vi "simpleReader.vi"() -> ()   [LabVIEW 2012]
uses:
  <userlib>/Common/Communication/ActiveMQ/ActiveMQBroker/ActiveMQBroker.lvclass
panel:
  out "messages received":string[][](table)
  in  "stopReader":bool
  in  "topic":string="testTopic"
  in  "port":string="61616"
  in  "host":string="localhost"
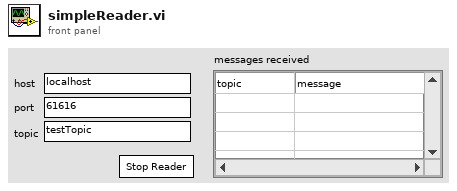
[diagram p1: front panel]
types:
  T1 = enum32{"invalid app kind", "Development System", "Run Time System", "Student Edition", "Embedded LabVIEW", "Evaluation", "Custom"}
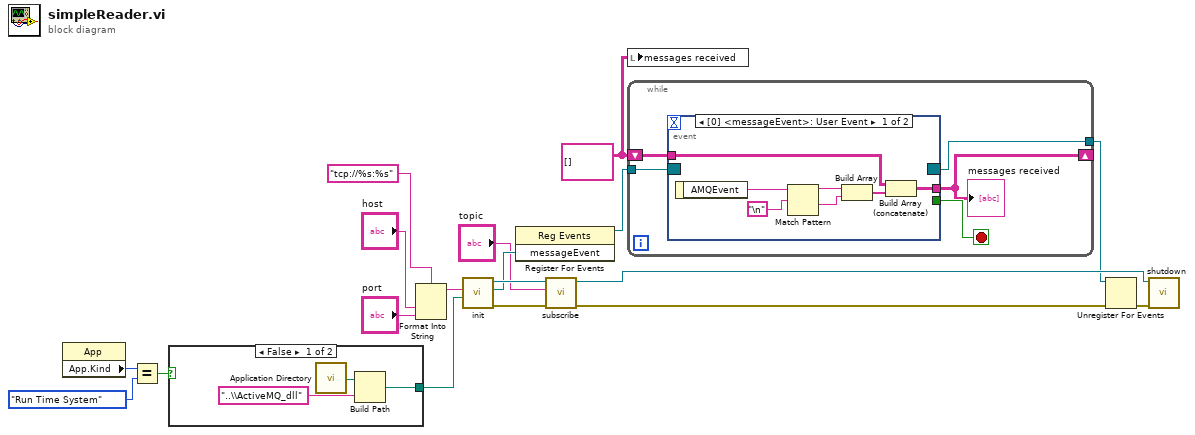
[diagram p0: block diagram]
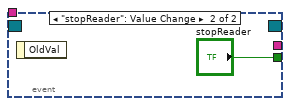
[diagram p2: hidden frame]
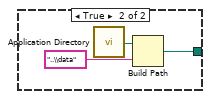
[diagram p3: hidden frame]
diagram:
  w1 = string[][] [] ("messages received")
  n1 = property class="App"() -> ("App.Kind"=w13:T1)  [unwired: 2 in, 2 out]
  n2 = Equal?(x=w13, y=T1."Run Time System") -> (x = y?=w11:bool)
  n3 = case shown="False" w11 {
    tunnel: [w19 w22] -> w18
    frame False {
      n4 = call <vilib>:"Application Directory.vi"() -> ("Application Directory"=w20:path)
      n5 = Build Path(base path=w20, name or relative path="..\\ActiveMQ_dll") -> (appended path=w19:path)
    }
    frame True {
      n6 = call <vilib>:"Application Directory.vi"() -> ("Application Directory"=w24:path)
      n7 = Build Path(base path=w24, name or relative path="..\\data") -> (appended path=w22:path)
    }
  }
  n8 = Format Into String(format string="tcp://%s:%s", "host", "port") -> (resulting string=w7:string)  [unwired: 2 in, 1 out]
  n9 = call <userlib>:"init.vi"("activeMQ_dll_directory"=w18, "brokerConnectionString"=w7) -> ("error out"=w17:errorcluster, "messageEvent"=w15:refnum<user-event>, "ActiveMQBroker out"=w16:refnum<class "ActiveMQBroker.lvclass">)  [unwired: 7 in]
  n10 = register-events(w15) -> (reference out=w6:refnum<event-registration>)  [unwired: 2 in, 1 out]
  n11 = call-dynamic "subscribe.vi"("error in (no error)"=w17, "source"="topic", "ActiveMQBroker in"=w16) -> ("error out"=w3:errorcluster, "ActiveMQBroker out"=w14:refnum<class "ActiveMQBroker.lvclass">)  [unwired: 7 in]
  n12 = local write "messages received"(w1) -> ()
  n13 = while {
    tunnel: w6 -> [w29]
    tunnel: [w28] -> w5
    shift-right: [w25] -> _
    shift-left: w1 -> [w27]
    stop <- w26 stop-if-true
    n14 = event shown="[0] <messageEvent>: User Event" {
      selector: w29 -> [_ _]
      dyn-events: [_ _] -> w28
      timeout: _ -> [_ _]
      tunnel: [w31 _] -> w25
      tunnel: w27 -> [w36 _]
      tunnel: [_ "stopReader"] -> w26
      event User Event {
        n15 = event-data() -> ("AMQEvent"=w35:string)  [unwired: 1 in]
        n16 = Match Pattern(string=w35, regular expression="\n") -> (before substring=w34:string, after substring=w33:string)  [unwired: 1 in, 2 out]
        n17 = Build Array(w34, w33) -> (w32:string[])
        n18 = Build Array (concatenate)(w36, w32) -> (w31:string[][])
      }
      event "stopReader": Value Change {
        n19 = event-data() -> ()  [unwired: 1 in, 1 out]
      }
    }
    "messages received" <- w25
  }
  n20 = Unregister For Events(event registration refnum=w5, error in=w3) -> (error out=w4:errorcluster)
  n21 = call-dynamic "shutdown.vi"("error in (no error)"=w4, "ActiveMQBroker in"=w14) -> ()  [unwired: 8 in, 2 out]
